vi "General Linear Fit (Bisquare).vi"(0 "Y":dbl[](array[numeric]), 1 "covariance selector":T3(ring), 5 "H":dbl[][](array[numeric]), 7 "Weight":dbl[](array[numeric]), 9 "tolerance":dbl=0.0001, 13 "algorithm":T1 items=["SVD", "Givens", "Givens2", "Householder", "LU Decomposition", "Cholesky", "SVD for Rank Deficient H"]) -> (4 "Best Fit":dbl[](array[numeric]), 6 "Coefficients":dbl[](array[numeric]), 8 "Covariance":T2, 10 "Weight Out":dbl[](array[numeric]), 14 "residue":dbl, 15 "error":i32)   [LabVIEW 2017, in "NI_AALPro.lvlib"]
uses:
  NI_AALPro.lvlib
  RealMatrix.ctl
  General Linear Fit Algorithm.ctl
  Array To Matrix - RA2.vi
  NI_Matrix.lvlib
  lvanlys.dll
panel:
  out "iteration":i32
  # "Bisquare General Linear Fit"
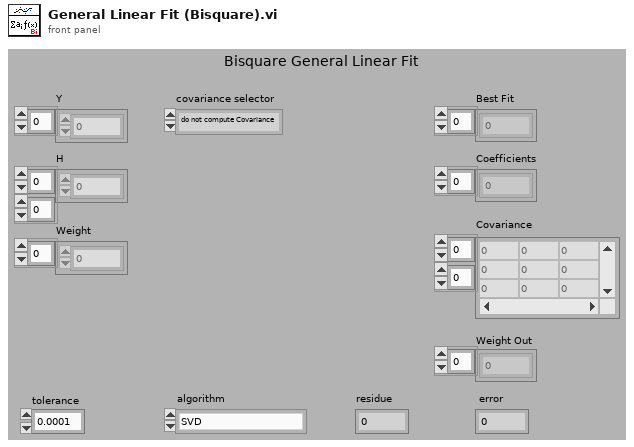
[diagram p1: front panel]
types:
  T1 = typedef "NI_AALPro.lvlib/General Linear Fit Algorithm.ctl" = u16
  T2 = typedef "NI_Matrix.lvlib/RealMatrix.ctl" = dbl[][]
  T3 = enum32{"do not compute Covariance", " compute Covariance"}
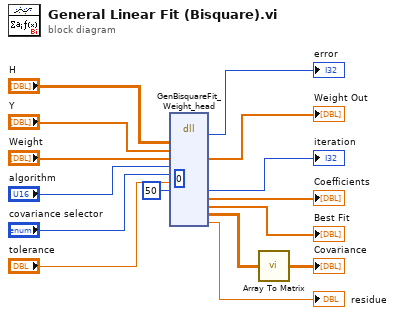
[diagram p0: block diagram]
diagram:
  (unwired) 0
  n1 = dll-call lib="C:/Program Files/National Instruments/LabVIEW 2017/resource/lvanlys.*" fn="GenBisquareFit_Weight_head" ("lvanlys.dll:GenBisquareFit_head")("H"="H", "Y Values"="Y", "Weight"="Weight", "algorithm"="algorithm", "covariance selector"="covariance selector", "tol"="tolerance", "maxIter"=50) -> ("return type"=→"error":i32, "Weight"=→"Weight Out":dbl[], "maxIter"=→"iteration":i32, "CoefH"=→"Coefficients":dbl[], "BestFitH"=→"Best Fit":dbl[], "CovarH"=w8:dbl[][], "mse"=→"residue":dbl)  [unwired: 7 in, 7 out]
  n2 = call-poly "Array To Matrix.vi"("Real 2D Array"=w8) -> ("Real Matrix"=→"Covariance":T2)
